vi "Reade.vi"(0 "Components type":string, 1 "ComponentsList":string, 2 "error in (no error)":errorcluster) -> (3 "To M Server":string, 4 "Address":string[][](array[string]), 5 "MD5":string, 6 "error out (no error)":errorcluster)   [LabVIEW 2011]
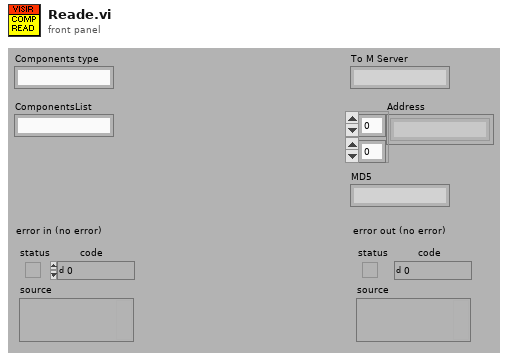
[diagram p1: front panel]
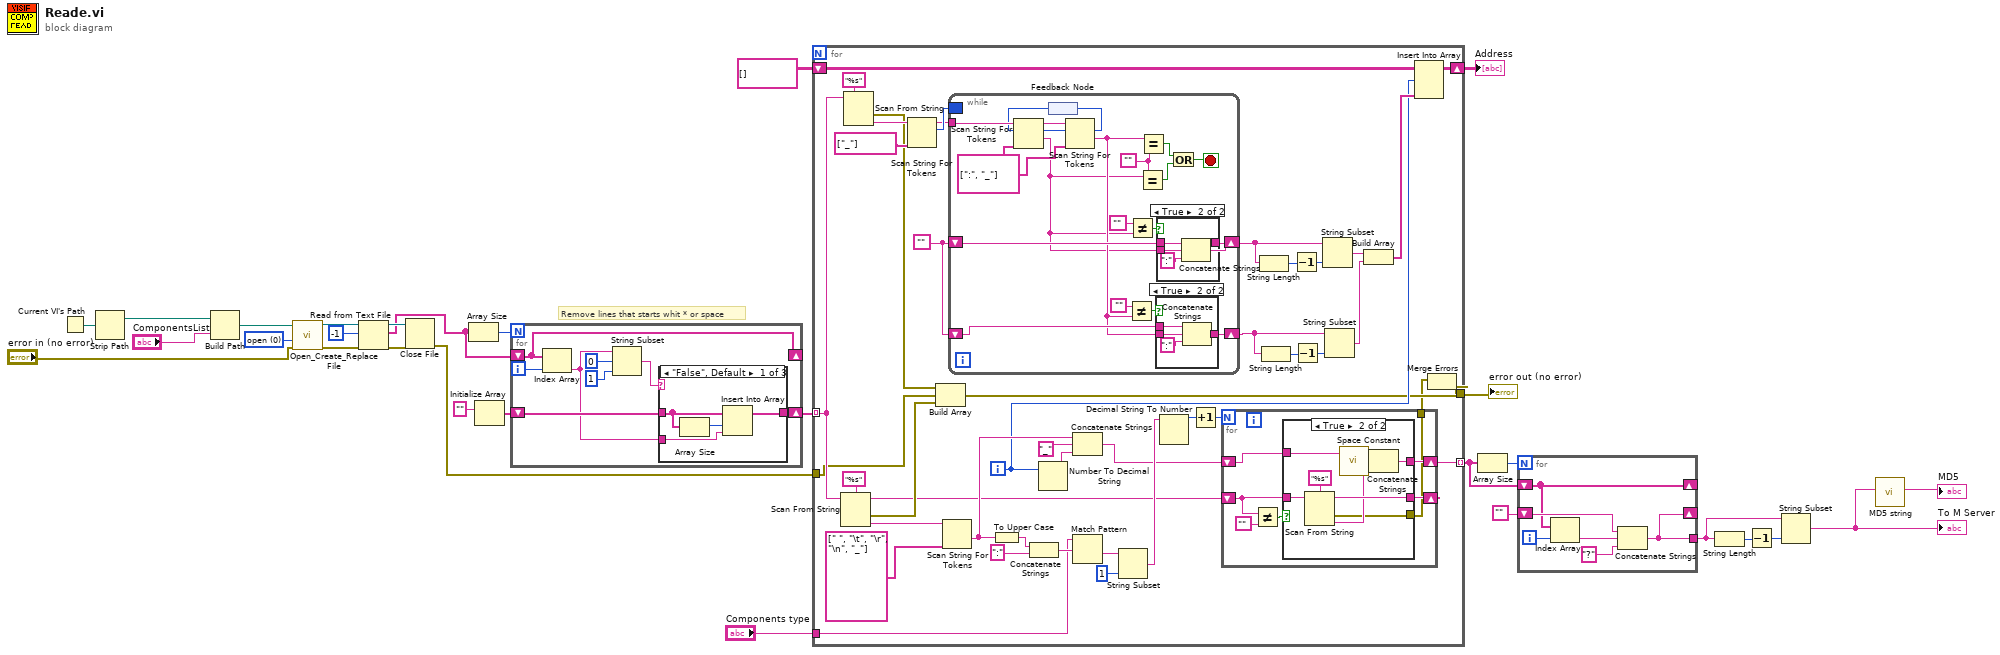
[diagram p0: block diagram]
diagram:
  w29 = i16 0 items=["open", "open or create", "create or replace", "create"] ("function")
  # "Remove lines that starts whit * or space"
  n1 = Current VI's Path() -> (path=w16:path)
  n2 = Strip Path(path=w16) -> (stripped path=w15:path)  [unwired: 1 out]
  n3 = Build Path(base path=w15, name or relative path="ComponentsList") -> (appended path=w14:path)
  n4 = call <vilib>:"Open_Create_Replace File.vi"("error in (no error)"="error in (no error)", "function (open:0)"=w29, "file path"=w14) -> ("error out"=w27:errorcluster, "refnum"=w28:refnum<file>)  [unwired: 5 in, 2 out]
  n5 = Read from Text File(file (use dialog)=w28, count=-1, error in=w27) -> (refnum out=w6:refnum<file>, text=w3:string[], error out=w5:errorcluster)  [unwired: 1 in, 1 out]
  n6 = Close File(refnum=w6, error in=w5) -> (error out=w4:errorcluster)  [unwired: 1 out]
  n7 = Array Size(array=w3) -> (size(s)=w8:i32)
  n8 = Initialize Array("") -> (w24:string[])  [unwired: 1 in]
  n9 = for {
    N: w8 -> [_]
    shift-right: [w33] -> _
    shift-left: w3 -> [w33]
    shift-right: [w31] -> w23
    shift-left: w24 -> [w32]
    i -> [w35]
    n10 = Index Array(array=w33, index=w35) -> (element=w30:string)
    n11 = String Subset(string=w30, offset (0)=0, length (rest)=1) -> (substring=w34:string)
    n12 = case shown="\"False\", Default" w34 {
      tunnel: w30 -> [w41 _ _]
      tunnel: w32 -> [w38 w42 w43]
      tunnel: [w39 w42 w43] -> w31
      frame "False", Default {
        n13 = Array Size(array=w38) -> (size(s)=w40:i32)
        n14 = Insert Into Array(array=w38, index=w40, new element=w41) -> (w39:string[])
      }
      frame "" {
      }
      frame "*" {
      }
    }
  }
  n15 = for {
    tunnel: w23 -> [w72] mode=indexing
    shift-right: [w65] -> w13
    shift-left: string[][] [] -> [w66]
    tunnel: [w45] -> w21 mode=indexing
    tunnel: "Components type" -> [w56]
    tunnel: w4 -> [w53]
    tunnel: [w51] -> w10
    i -> [w74]
    w67 = ""
    n16 = Scan From String(format string="%s", input string=w72) -> (remaining string=w49:string, error out=w54:errorcluster, output 1=w85:string)  [unwired: 3 in, 1 out]
    n17 = Scan From String(format string="%s", input string=w72) -> (error out=w55:errorcluster, output 1=w69:string)  [unwired: 3 in, 2 out]
    n18 = Scan String For Tokens(6:string[] ["_"], 9:w69) -> (2:w70:i32, 3:w68:string)  [unwired: 4 in, 2 out]
    n19 = Build Array(w55, w53, w54) -> (w52:errorcluster[])
    n20 = Scan String For Tokens(6:string[] [" ", "\t", "\r", "\n", "_"], 9:w85) -> (1:w76:string)  [unwired: 4 in, 3 out]
    n21 = while {
      tunnel: w68 -> [w121]
      shift-right: [w105] -> w61
      shift-left: w67 -> [w113]
      shift-right: [w106] -> w57
      shift-left: w67 -> [w112]
      border: w70 -> [_]
      stop <- w115 stop-if-true
      w118 = ""
      w114 = string[] [":", "_"]
      n22 = feedback #1() -> (w120:i32)
      n23 = Scan String For Tokens(6:w114, 8:w120, 9:w121) -> (1:w104:string, 2:w119:i32, 3:w122:string)  [unwired: 3 in, 1 out]
      n24 = Scan String For Tokens(6:w114, 8:w119, 9:w122) -> (1:w107:string, 2:w123:i32)  [unwired: 3 in, 2 out]
      n25 = feedback-in #1(w123) -> ()
      n26 = Not Equal?(x="", y=w107) -> (x != y?=w108:bool)
      n27 = Not Equal?(x="", y=w104) -> (x != y?=w111:bool)
      n28 = Equal?(x=w104, y=w118) -> (x = y?=w116:bool)
      n29 = Equal?(x=w107, y=w118) -> (x = y?=w117:bool)
      n30 = case shown="True" w108 {
        tunnel: w107 -> [_ w127]
        tunnel: [w124 w126] -> w106
        tunnel: w112 -> [w124 w125]
        frame False {
        }
        frame True {
          n31 = Concatenate Strings(w125, w127, ":") -> (w126:string)
        }
      }
      n32 = case shown="True" w111 {
        tunnel: w104 -> [_ w132]
        tunnel: w113 -> [w129 w131]
        tunnel: [w129 w130] -> w105
        frame False {
        }
        frame True {
          n33 = Concatenate Strings(w131, w132, ":") -> (w130:string)
        }
      }
      n34 = Or(x=w117, y=w116) -> (x .or. y?=w115:bool)
    }
    n35 = To Upper Case(1:w76) -> (0:w77:string)
    n36 = Concatenate Strings(w77, ":") -> (w82:string)
    n37 = Number To Decimal String(number=w74) -> (decimal integer string=w81:string)  [unwired: 1 in]
    n38 = Concatenate Strings(w76, "_", w81) -> (w48:string)
    n39 = Match Pattern(string=w56, regular expression=w82) -> (after substring=w79:string)  [unwired: 1 in, 3 out]
    n40 = String Subset(string=w79, length (rest)=1) -> (substring=w50:string)  [unwired: 1 in]
    n41 = Decimal String To Number(string=w50) -> (number=w46:i32)  [unwired: 2 in, 1 out]
    n42 = Increment(x=w46) -> (x+1=w47:i32)
    n43 = for {
      N: w47 -> [_]
      shift-right: [w93] -> _
      shift-left: w49 -> [w91]
      shift-right: [w88] -> w45
      shift-left: w48 -> [w89]
      tunnel: [w87] -> w44
      n44 = Not Equal?(x=w91, y="") -> (x != y?=w92:bool)
      n45 = case shown="True" w92 {
        tunnel: w91 -> [w95 w102]
        tunnel: [w95 w101] -> w93
        tunnel: w89 -> [w94 w98]
        tunnel: [w94 w97] -> w88
        tunnel: [_ w96] -> w87
        frame False {
        }
        frame True {
          n46 = Scan From String(format string="%s", input string=w102) -> (remaining string=w101:string, error out=w96:errorcluster, output 1=w99:string)  [unwired: 3 in, 1 out]
          n47 = call <vilib>:"Space Constant.vi"() -> ("String"=w100:string)
          n48 = Concatenate Strings(w98, w100, w99) -> (w97:string)
        }
      }
    }
    n49 = String Length(string=w61) -> (length=w63:i32)
    n50 = String Length(string=w57) -> (length=w59:i32)
    n51 = Decrement(x=w63) -> (x-1=w64:i32)
    n52 = Decrement(x=w59) -> (x-1=w60:i32)
    n53 = String Subset(string=w61, length (rest)=w64) -> (substring=w62:string)  [unwired: 1 in]
    n54 = String Subset(string=w57, length (rest)=w60) -> (substring=w58:string)  [unwired: 1 in]
    n55 = Build Array(w62, w58) -> (w75:string[])
    n56 = Insert Into Array(array=w66, index (row)=w74, new element=w75) -> (w65:string[][])  [unwired: 1 in]
    n57 = Merge Errors(w44, w52) -> (w51:errorcluster)
  }
  "Address" <- w13
  "error out (no error)" <- w10
  n58 = Array Size(array=w21) -> (size(s)=w7:i32)
  n59 = for {
    N: w7 -> [_]
    shift-right: [w134] -> _
    shift-left: w21 -> [w134]
    tunnel: [w135] -> w17
    shift-right: [w135] -> _
    shift-left: "" -> [w138]
    i -> [w139]
    n60 = Index Array(array=w134, index=w139) -> (element=w137:string)
    n61 = Concatenate Strings(w138, w137, "?") -> (w135:string)
  }
  n62 = String Length(string=w17) -> (length=w19:i32)
  n63 = Decrement(x=w19) -> (x-1=w18:i32)
  n64 = String Subset(string=w17, length (rest)=w18) -> (substring=w2:string)  [unwired: 1 in]
  "To M Server" <- w2
  n65 = call "MD5 string.vi"("Message String"=w2) -> ("MD5 message-digest"=→"MD5":string)  [unwired: 10 in]
